vi "zmq_recv_multi.vi"(3 "error in":errorcluster, 5 "socket in":refnum<class "zmq_socket.lvclass">) -> (0 "error out":errorcluster, 1 "parts":string[](array[string]), 2 "socket out":refnum<class "zmq_socket.lvclass">)   [LabVIEW 2020, in "zeromq.lvlib" / "zmq_socket.lvclass"]
doc: "Receive a multi-component message from the socket. The incoming messages are returned as an array of strings, with one string for each message part.\n\nIf <b>no block?</b> is True, the function call will return immediately. Use zmq_check_timeout to see if it was simply a timeout or an error occurred.\n\nOtherwise this call will block until <b>all</b> parts of the message are received, an error is raised, or the socket is closed.\n\nNote there is no penalty using this function to receive single-part messages.\n\nDetailed API documentation: http://api.zeromq.org/3-2:zmq-recv"
uses:
  zmq_socket.lvclass
  zmq_socket.lvclass/zmq_socket.ctl
  Error Cluster From Error Code.vi
  zeromq.lvlib
panel:
  # "ØMQ"
  # "labview"
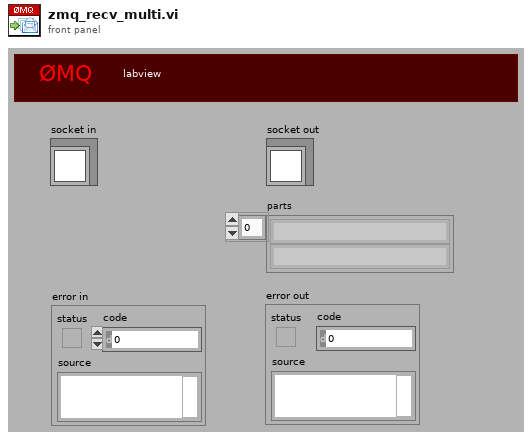
[diagram p1: front panel]
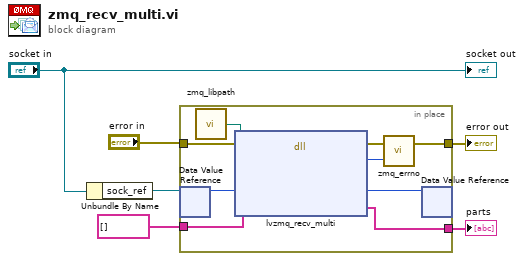
[diagram p0: block diagram]
diagram:
  n1 = Unbundle By Name("socket in") -> ("sock_ref"=w2:refnum<data-value>)
  n2 = in-place {
    in-place-border: "error in" -> [w13]
    in-place-border: [w12] -> w5
    in-place-border: string[] [] ("parts") -> [w11]
    in-place-border: [w8] -> w1
    n3 = in-place-dvr #1(w2) -> (w10:u64)  [unwired: 1 out]
    n4 = call "zmq_libpath.vi"() -> ("path"=w7:path)
    n5 = dll-call lib="?" fn="lvzmq_recv_multi" ("zmq_labview.dll:lvzmq_socket")(path in=w7, error in=w13, "sock_obj"=w10, "data"=w11) -> (error out=w15:errorcluster, "return type"=w14:i32, "sock_obj"=w9:u64, "data"=w8:string[])  [unwired: 3 in, 1 out]
    n6 = call "zmq_errno.vi"("retval"=w14, "error in"=w15) -> ("error out"=w12:errorcluster)  [unwired: 1 out]
    n7 = in-place-dvr #1(w9) -> ()  [unwired: 2 out]
  }
  "error out" <- w5
  "parts" <- w1
  "socket out" <- "socket in"
